vi "UserGuide-DataAcquire.vi"() -> ()   [LabVIEW 2016]
panel:
  out "Caller":string
  out "字符串":string
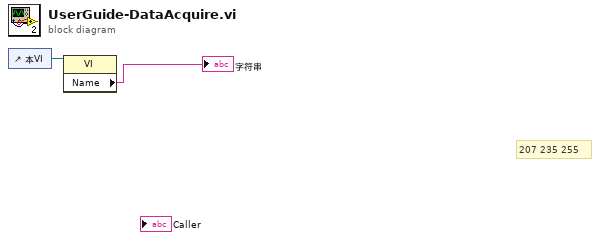
[diagram p0: block diagram]
diagram:
  # "207 235 255"
  n1 = control-ref of="本VI"() -> (w2:refnum<vi>)
  n2 = property class="VI"(reference=w2) -> ("Name"=→"字符串":string)  [unwired: 1 in, 2 out]
